vi "NAV.vi"(0 "System no.":i32=1 min=1 max=4 step=1, 1 "Board":i32=1 min=1 max=5 step=1, 3 "Number of \nreadings":i16=1 min=0 max=20 step=1, 5 "error in":errorcluster) -> (14 "Controller error":bool, 19 "error out":errorcluster)   [LabVIEW 2020]
doc: "Sets averaging count for analog readings. Controller error is TRUE if selected system reports an error code which is not 0. For large count values, the communication timeout value may need to be increased to prevent a timeout error during TAV? queries."
uses:
  Syntax.ctl
  Global1.vi
panel:
  # "Sets averaging count for analog readings. For large count\nvalues the communication timeout value may need to be\nincreased to prevent a timeout during TAV? queries."
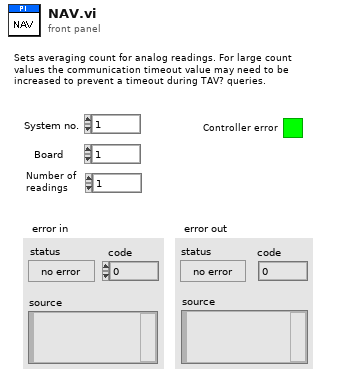
[diagram p1: front panel]
types:
  T1 = typedef "Syntax.ctl" = enum16{"GCS 1.0", "GCS 2.0", "GCS 3.0"}
  T2 = enum16{"Disable error check", "Force error check", "Use global settings"}
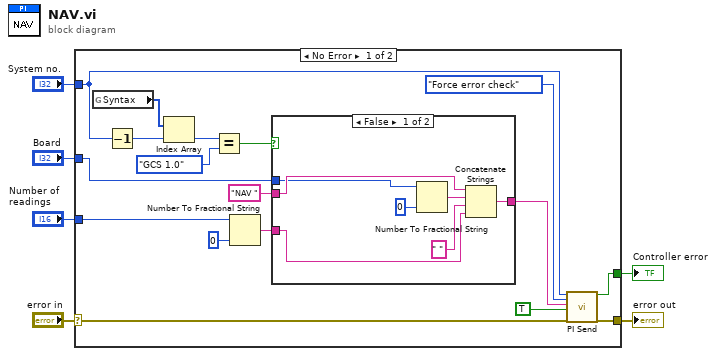
[diagram p0: block diagram]
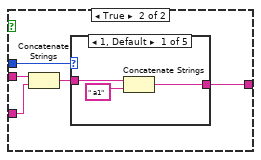
[diagram p2: hidden frame]
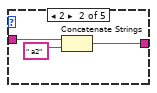
[diagram p3: hidden frame]
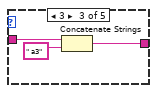
[diagram p4: hidden frame]
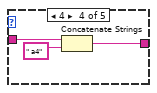
[diagram p5: hidden frame]
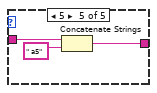
[diagram p6: hidden frame]
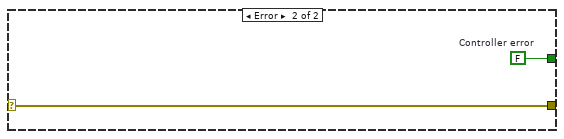
[diagram p7: hidden frame]
diagram:
  n1 = case shown="No Error" "error in" {
    selector: "error in" -> [w11 w52]
    tunnel: [w9 w52] -> w6
    tunnel: [w10 w51] -> w5
    tunnel: "Number of \nreadings" -> [w22 _]
    tunnel: "Board" -> [w18 _]
    tunnel: "System no." -> [w15 _]
    frame No Error {
      n2 = global read "Global1.vi" "Syntax"() -> (w16:T1[])
      n3 = Decrement(x=w15) -> (x-1=w14:i32)
      n4 = Index Array(array=w16, index=w14) -> (element=w13:T1)
      n5 = Equal?(x=w13, y=Syntax."GCS 1.0") -> (x = y?=w12:bool)
      n6 = Number To Fractional String(number=w22, precision (6)=i16 0) -> (F-format string=w21:string)  [unwired: 2 out]
      n7 = case shown="False" w12 {
        tunnel: "NAV " -> [w30 w35]
        tunnel: w21 -> [w25 w34]
        tunnel: w18 -> [w28 w33]
        tunnel: [w24 w32] -> w17
        frame False {
          n8 = Number To Fractional String(number=w28, precision (6)=i16 0) -> (F-format string=w27:string)  [unwired: 2 out]
          n9 = Concatenate Strings(w30, w27, " ", w25) -> (w24:string)
        }
        frame True {
          n10 = Concatenate Strings(w35, w34) -> (w31:string)
          n11 = case shown="1, Default" w33 {
            tunnel: w31 -> [w38 w41 w44 w47 w50]
            tunnel: [w36 w39 w42 w45 w48] -> w32
            frame 1, Default {
              n12 = Concatenate Strings(w38, " a1" ("Substring")) -> (w36:string)
            }
            frame 2 {
              n13 = Concatenate Strings(w41, " a2" ("Substring")) -> (w39:string)
            }
            frame 3 {
              n14 = Concatenate Strings(w44, " a3" ("Substring")) -> (w42:string)
            }
            frame 4 {
              n15 = Concatenate Strings(w47, " a4" ("Substring")) -> (w45:string)
            }
            frame 5 {
              n16 = Concatenate Strings(w50, " a5" ("Substring")) -> (w48:string)
            }
          }
        }
      }
      n17 = call "PI Send.vi"("System no."=w15, "Error check settings"=T2."Force error check", "String to send"=w17, "Attach termination char.?"=TRUE ("Attach Linefeed?"), "error in"=w11) -> ("Controller error"=w10:bool, "error out"=w9:errorcluster)  [unwired: 1 in, 12 out]
    }
    frame Error {
      w51 = FALSE  # Controller error
    }
  }
  "error out" <- w6
  "Controller error" <- w5
